vi "Sequence Default New.vi"(1 "Username":string, 2 "Post Data":T1) -> (0 "Default New Instrument":T2)   [LabVIEW 2011]
uses:
  Sequence Record.ctl
  Addons/internet/utils/keyedarr.llb/Keyed Array.ctl
  Addons/internet/utils/strutil.llb/Case Matching.ctl
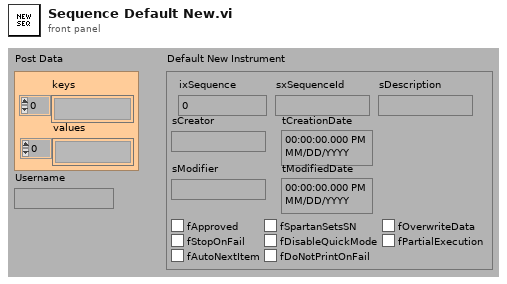
[diagram p1: front panel]
types:
  T1 = typedef "Keyed Array.ctl" = cluster{"keys":string[], "values":string[]}
  T2 = typedef "Sequence Record.ctl" = cluster{"ixSequence":i32, "sxSequenceId":string, "sDescription":string, "sCreator":string, "tCreationDate":timestamp, "sModifier":string, "tModifiedDate":timestamp, "fApproved":bool, "fSpartanSetsSN":bool, "fOverwriteData":bool, "fStopOnFail":bool, "fDisableQuickMode":bool, "fPartialExecution":bool, "fAutoNextItem":bool, "fDoNotPrintOnFail":bool}
  T3 = typedef "Case Matching.ctl" = enum16{"a != A", "a == A", "system"}
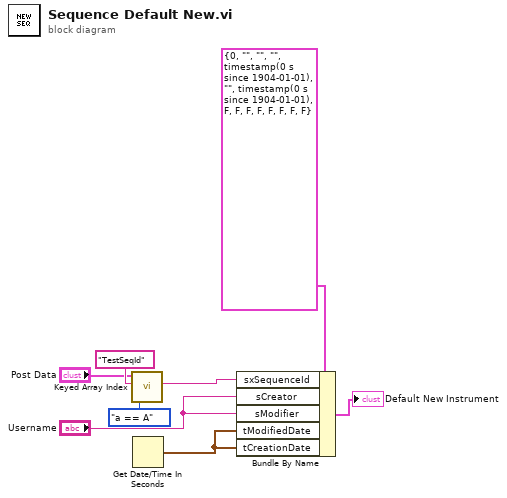
[diagram p0: block diagram]
diagram:
  n1 = call "Keyed Array Index.vi"("case matching (sensitive)"=Case_Matching."a == A", "key"="TestSeqId", "array in"="Post Data") -> ("value"=w3:string)  [unwired: 1 in, 3 out]
  n2 = Get Date/Time In Seconds() -> (seconds since 1Jan1904=w1:timestamp)
  n3 = Bundle By Name(cluster=T2 {"ixSequence"=0, "sxSequenceId"="", "sDescription"="", "sCreator"="", "tCreationDate"=timestamp(0 s since 1904-01-01), "sModifier"="", "tModifiedDate"=timestamp(0 s since 1904-01-01), "fApproved"=FALSE, "fSpartanSetsSN"=FALSE, "fOverwriteData"=FALSE, "fStopOnFail"=FALSE, "fDisableQuickMode"=FALSE, "fPartialExecution"=FALSE, "fAutoNextItem"=FALSE, "fDoNotPrintOnFail"=FALSE} ("Default New Instrument"), "sxSequenceId"=w3, "sCreator"="Username", "sModifier"="Username", "tModifiedDate"=w1, "tCreationDate"=w1) -> (→"Default New Instrument":T2)
